vi "GetCurrentTime.vi"(5 "Date Operation (Get)":enum16{"Get", "None (Future)"}(ring), 6 "error constant":errorcluster, 7 "Event Information":cluster{string, string}={"Boiler Initialize", "0"}, 8 "want seconds? (F)":bool=TRUE, 9 "date format (0)":enum16{"short", "long", "abbreviated"}(ring)) -> (0 "error IO":errorcluster, 2 "Cluster":cluster{string, string}, 3 "Array":string[](array[string]))   [LabVIEW 2016]
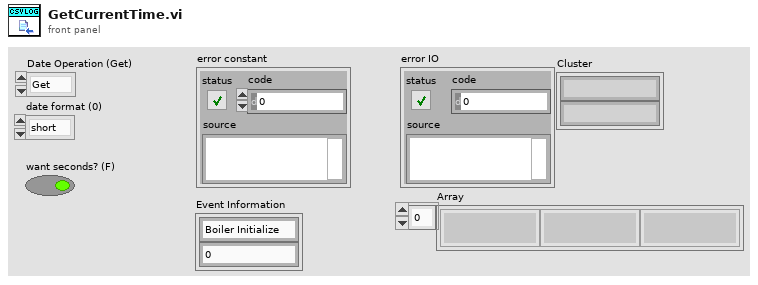
[diagram p1: front panel]
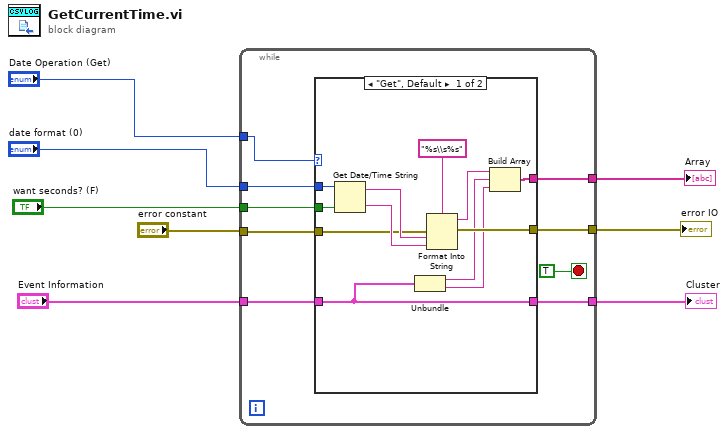
[diagram p0: block diagram]
diagram:
  n1 = while {
    tunnel: "Date Operation (Get)" -> [w16]
    tunnel: "date format (0)" -> [w15]
    tunnel: "want seconds? (F)" -> [w14]
    tunnel: "error constant" -> [w13]
    tunnel: [w12] -> w4
    tunnel: [w11] -> w3
    tunnel: "Event Information" -> [w10]
    tunnel: [w9] -> w1
    stop <- TRUE stop-if-true
    n2 = case shown="\"Get\", Default" w16 {
      tunnel: w15 -> [w26 _]
      tunnel: w14 -> [w25 _]
      tunnel: w13 -> [w24 w31]
      tunnel: [w23 w31] -> w12
      tunnel: [w22 _] -> w11
      tunnel: w10 -> [w18 w30]
      tunnel: [w18 w30] -> w9
      frame "Get", Default {
        n3 = Get Date/Time String(date format (0)=w26, want seconds? (F)=w25) -> (date string=w29:string, time string=w28:string)  [unwired: 1 in]
        n4 = Unbundle(w18) -> (w20:string, w19:string)
        n5 = Format Into String(format string="%s\\s%s", error in=w24, w29, w28) -> (resulting string=w21:string, error out=w23:errorcluster)  [unwired: 1 in]
        n6 = Build Array(w21, w20, w19) -> (w22:string[])
      }
      frame "None (Future)" {
      }
    }
  }
  "error IO" <- w4
  "Array" <- w3
  "Cluster" <- w1
